vi "Bundle control and indicator references.vi"(8 "error in":errorcluster, 11 "UI elements cluster":T2) -> (0 "error out":errorcluster, 3 "UI elements cluster":T2)   [LabVIEW 2020]
uses:
  Typedefs/UI ctrl refs cluster.ctl
  Typedefs/Laser control knob.ctl
  Typedefs/Frame Size.ctl
  Typedefs/Plane Mode.ctl
  Typedefs/PMT control knob.ctl
  Typedefs/XY Stage_Move.ctl
  Typedefs/test_fpga_control.ctl
  Acquisition/Typedefs/Ref DAQ Param.ctl
  Experiment Type.ctl
  Biology Information.ctl
  Global Variables/gl_UI Ctrl Refs.vi
panel:
  out "Cluster":T1
  in  "RefDAQParam 2":refnum<vi>
  out "Ctrl ref names in typedef cluster":string[](array[string])
  out "Dynamically acquired UI element names":string[](array[string])
  out "Errors":errorcluster[](array[cluster])
  out "UI element names and status":cluster{"Label.Text":string, "Found":bool}[](array[cluster])
  # "<----- If the LED is off for a UI element it means that that this VI fails to acquire its reference correctly. In that case upgrade this VI to handle that element."
  # "The top 5 should be the same.\nThe rest should be updated so not the same."
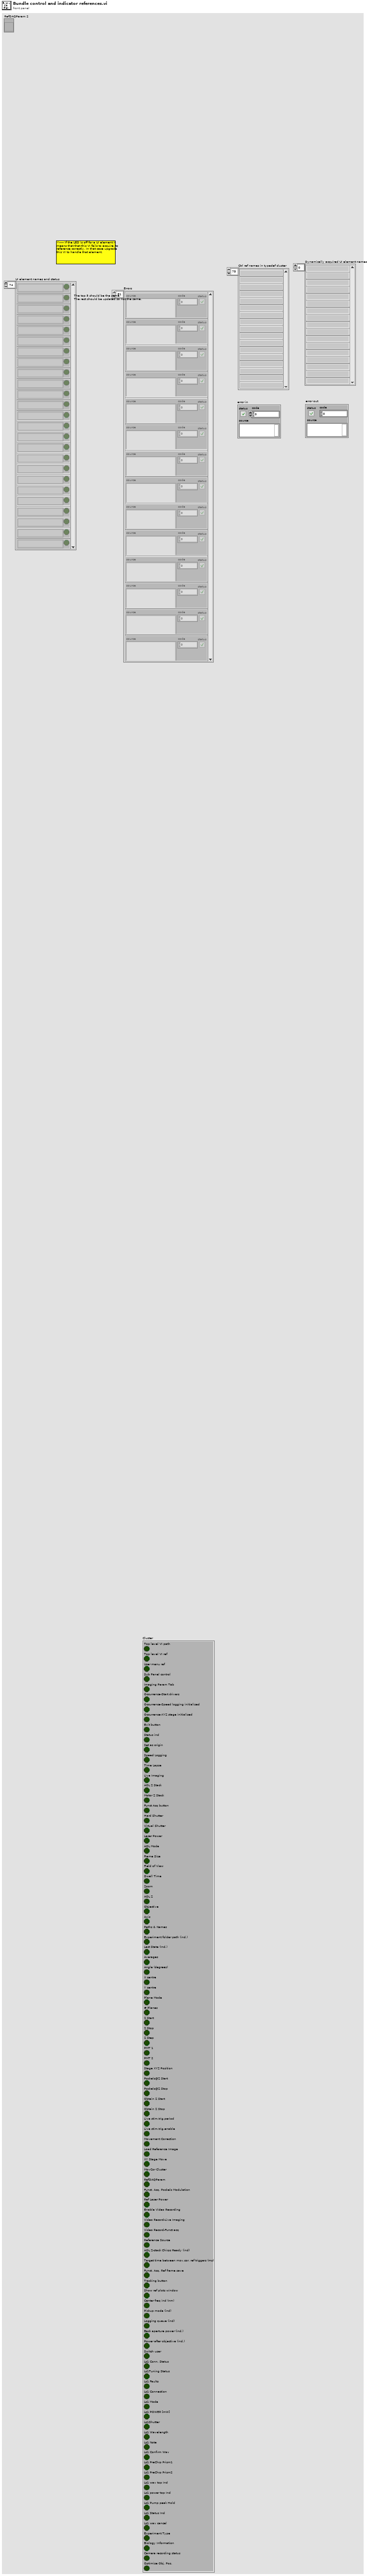
[diagram p1: front panel]
types:
  T1 = cluster{"Top level VI path":bool, "Top level VI ref":bool, "User menu ref":bool, "Sub Panel control":bool, "Imaging Param Tab":bool, "Occurrence-Start drivers":bool, "Occurrence-Speed logging initialised":bool, "Occurrence-XYZ stage initialised":bool, "Exit button":bool, "Status ind":bool, "Set as origin":bool, "Speed Logging":bool, "Time Lapse":bool, "Live Imaging":bool, "AOL Z Stack":bool, "Motor Z Stack":bool, "Funct Acq button":bool, "Hard Shutter":bool, "Virtual Shutter":bool, "Laser Power":bool, "AOL Mode":bool, "Frame Size":bool, "Field of View":bool, "Dwell Time":bool, "Zoom":bool, "AOL Z":bool, "Objective":bool, "Axis":bool, "Paths & Names":bool, "Experiment folder path (ind.)":bool, "Last State (Ind.)":bool, "Averages":bool, "Angle (degrees)":bool, "X centre":bool, "Y centre":bool, "Plane Mode":bool, "# Planes":bool, "Z Start":bool, "Z Stop":bool, "Z Step":bool, "PMT 1":bool, "PMT 2":bool, "Stage XYZ Position":bool, "Pockels@Z Start":bool, "Pockels@Z Stop":bool, "Obtain Z Start":bool, "Obtain Z Stop":bool, "Live stim.trig.period":bool, "Live stim.trig.enable":bool, "Movement Correction":bool, "Load Reference Image":bool, "XY Stage Move":bool, "MovCor Cluster":bool, "RefDAQParam":bool, "Funct. Acq. Pockels Modulation":bool, "Ref Laser Power":bool, "Enable Video Recording":bool, "Video Record-Live Imaging":bool, "Video Record-Funct acq":bool, "Reference Source":bool, "AOL Z-stack Chirps Ready (ind)":bool, "Target time between mov.cor. ref triggers (ms)":bool, "Funct. Acq. Ref frame save":bool, "Tracking button":bool, "Show ref plots window":bool, "Center freq ind (nm)":bool, "Pickup mode (ind)":bool, "Logging queue (ind)":bool, "Back aperture power (ind.)":bool, "Power after objective (ind.)":bool, "Switch user":bool, "Ls1 Conn. Status":bool, "Ls1Tuning Status":bool, "Ls1 Faults":bool, "Ls1 Connection":bool, "Ls1 Mode":bool, "Ls1 POWER [mW]":bool, "Ls1Shutter":bool, "Ls1 Wavelength":bool, "Ls1 Note":bool, "Ls1 Confirm Wav":bool, "Ls1 PreChrp Prism1":bool, "Ls1 PreChrp Prism2":bool, "Ls1 wav top Ind":bool, "Ls1 power top Ind":bool, "Ls1 Pump peak Hold":bool, "Ls1 Status Ind":bool, "Ls1 wav cancel":bool, "Experiment Type":bool, "Biology Information":bool, "Camera recording status":bool, "Optimise Obj. Pos.":bool}
  T2 = typedef "UI ctrl refs cluster.ctl" = cluster{"Top level VI path":path, "Top level VI ref":refnum<vi>, "User menu ref":refnum<k9>, "Sub Panel control":refnum<vi>, "Imaging Param Tab":refnum<vi>, "Occurrence-Start drivers":refnum<k4>, "Occurrence-Speed logging initialised":refnum<k4>, "Occurrence-XYZ stage initialised":refnum<k4>, "Exit button":refnum<vi>, "Status ind":refnum<vi>, "Set as origin":refnum<vi>, "Speed Logging":refnum<vi>, "Time Lapse":refnum<vi>, "Live Imaging":refnum<vi>, "AOL Z Stack":refnum<vi>, "Motor Z Stack":refnum<vi>, "Funct Acq button":refnum<vi>, "Hard Shutter":refnum<vi>, "Virtual Shutter":refnum<vi>, "Laser Power":refnum<vi>, "AOL Mode":refnum<vi>, "Frame Size":refnum<vi>, "Field of View":refnum<vi>, "Dwell Time":refnum<vi>, "Zoom":refnum<vi>, "AOL Z":refnum<vi>, "Objective":refnum<vi>, "Axis":refnum<vi>, "Paths & Names":refnum<vi>, "Experiment folder path (ind.)":refnum<vi>, "Last State (Ind.)":refnum<vi>, "Averages":refnum<vi>, "Angle (degrees)":refnum<vi>, "X centre":refnum<vi>, "Y centre":refnum<vi>, "Plane Mode":refnum<vi>, "# Planes":refnum<vi>, "Z Start":refnum<vi>, "Z Stop":refnum<vi>, "Z Step":refnum<vi>, "PMT 1":refnum<vi>, "PMT 2":refnum<vi>, "Stage XYZ Position":refnum<vi>, "Pockels@Z Start":refnum<vi>, "Pockels@Z Stop":refnum<vi>, "Obtain Z Start":refnum<vi>, "Obtain Z Stop":refnum<vi>, "Live stim.trig.period":refnum<vi>, "Live stim.trig.enable":refnum<vi>, "Movement Correction":refnum<vi>, "Load Reference Image":refnum<vi>, "XY Stage Move":refnum<vi>, "MovCor Cluster":refnum<vi>, "RefDAQParam":refnum<vi>, "Funct. Acq. Pockels Modulation":refnum<vi>, "Ref Laser Power":refnum<vi>, "Enable Video Recording":refnum<vi>, "Video Record-Live Imaging":refnum<vi>, "Video Record-Funct acq":refnum<vi>, "Reference Source":refnum<vi>, "AOL Z-stack Chirps Ready (ind)":refnum<vi>, "Target time between mov.cor. ref triggers (ms)":refnum<vi>, "Funct. Acq. Ref frame save":refnum<vi>, "Tracking button":refnum<vi>, "Show ref plots window":refnum<vi>, "Center freq ind (nm)":refnum<vi>, "Pickup mode (ind)":refnum<vi>, "Logging queue (ind)":refnum<vi>, "Back aperture power (ind.)":refnum<vi>, "Power after objective (ind.)":refnum<vi>, "Switch user":refnum<vi>, "Ls1 Conn. Status":refnum<vi>, "Ls1Tuning Status":refnum<vi>, "Ls1 Faults":refnum<vi>, "Ls1 Connection":refnum<vi>, "Ls1 Mode":refnum<vi>, "Ls1 POWER [mW]":refnum<vi>, "Ls1Shutter":refnum<vi>, "Ls1 Wavelength":refnum<vi>, "Ls1 Note":refnum<vi>, "Ls1 Confirm Wav":refnum<vi>, "Ls1 PreChrp Prism1":refnum<vi>, "Ls1 PreChrp Prism2":refnum<vi>, "Ls1 wav top Ind":refnum<vi>, "Ls1 power top Ind":refnum<vi>, "Ls1 Pump peak Hold":refnum<vi>, "Ls1 Status Ind":refnum<vi>, "Ls1 wav cancel":refnum<vi>, "Experiment Type":refnum<vi>, "Biology Information":refnum<vi>, "Camera recording status":refnum<vi>, "Optimise Obj. Pos.":refnum<vi>}
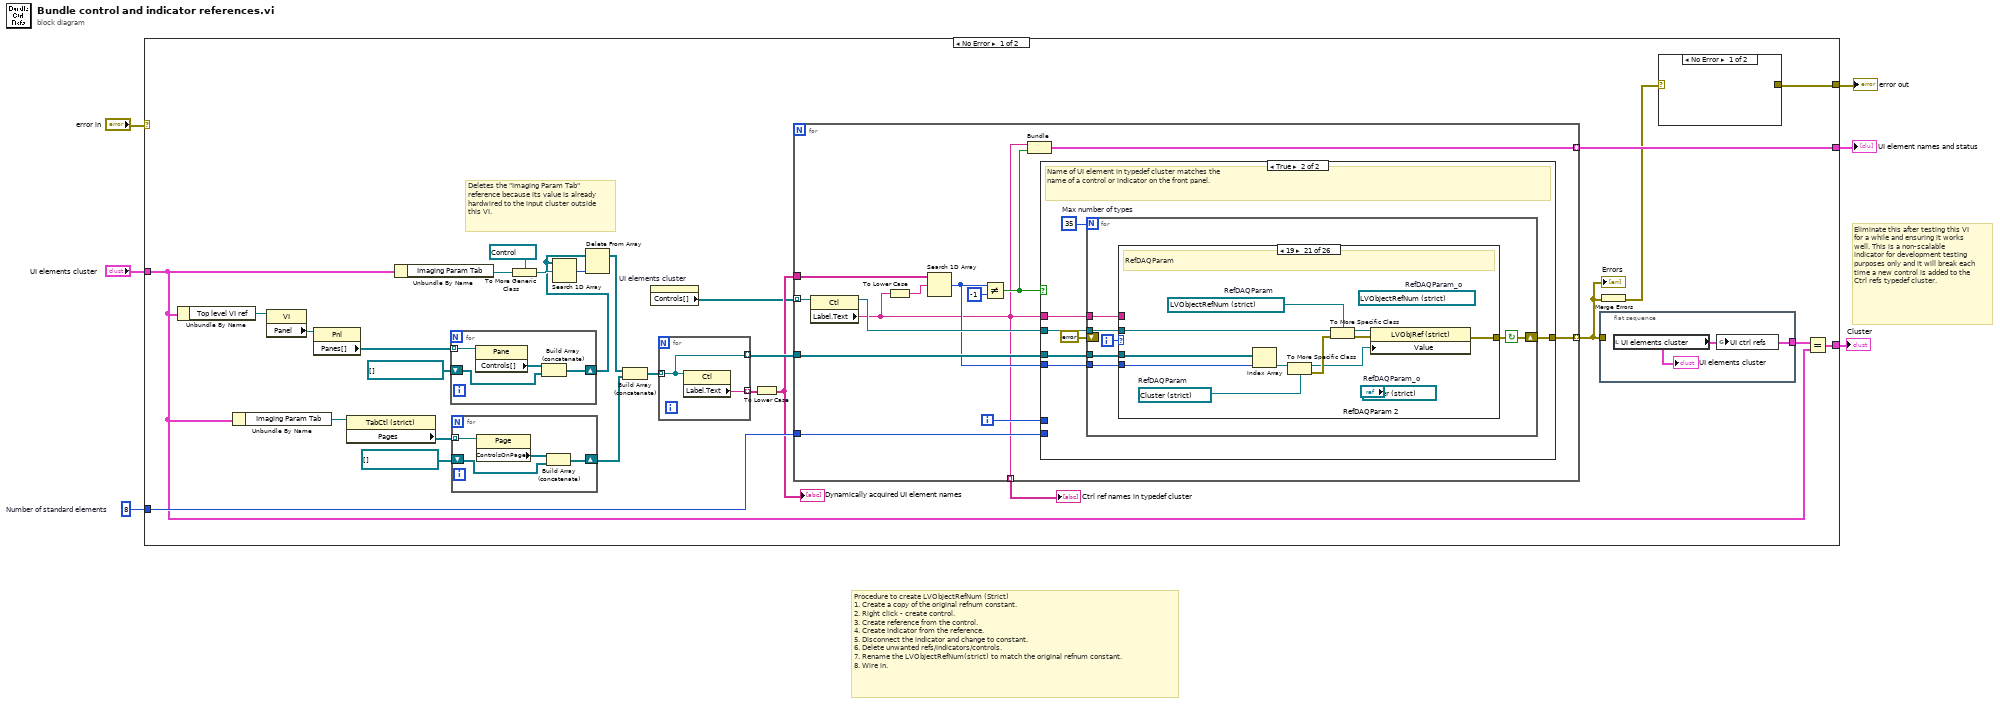
[diagram p0: block diagram]
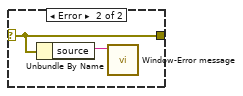
[diagram p2: hidden frame]
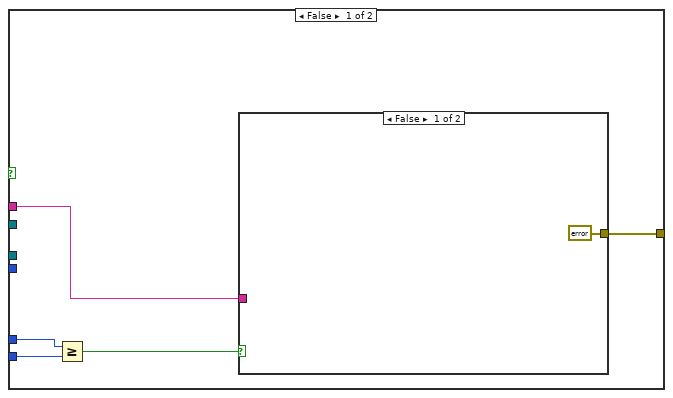
[diagram p3: hidden frame]
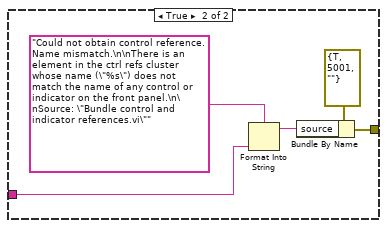
[diagram p4: hidden frame]
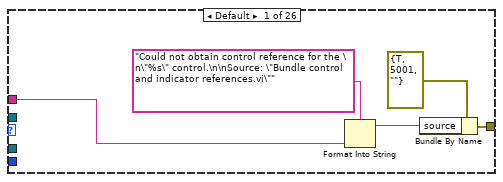
[diagram p5: hidden frame]
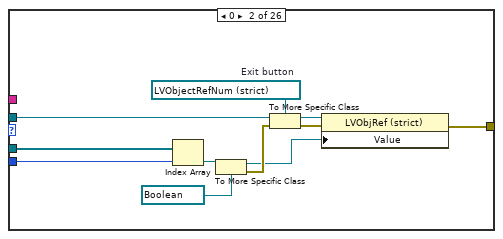
[diagram p6: hidden frame]
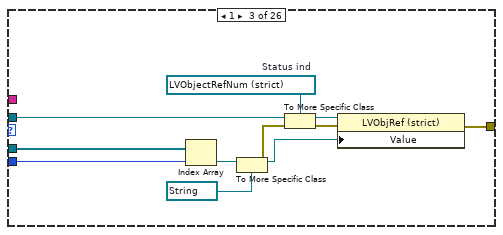
[diagram p7: hidden frame]
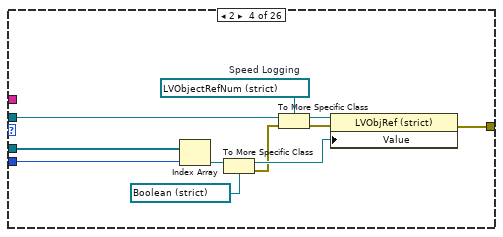
[diagram p8: hidden frame]
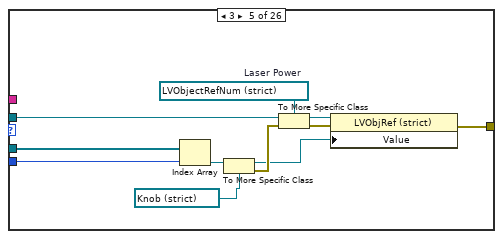
[diagram p9: hidden frame]
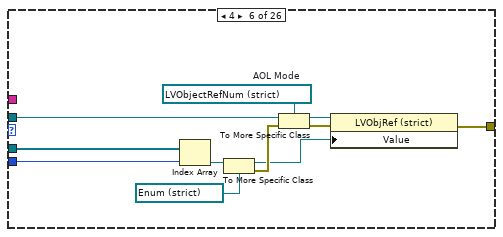
[diagram p10: hidden frame]
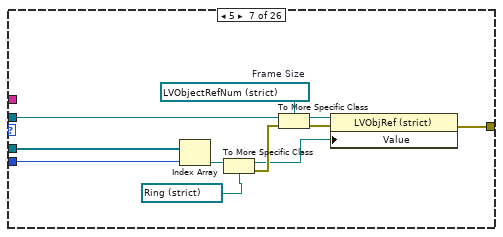
[diagram p11: hidden frame]
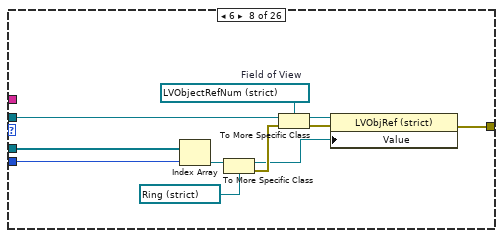
[diagram p12: hidden frame]
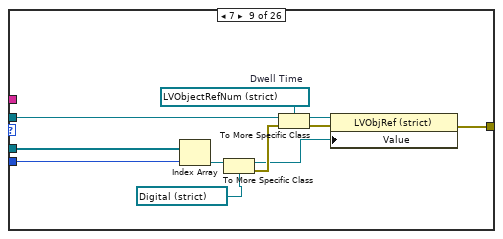
[diagram p13: hidden frame]
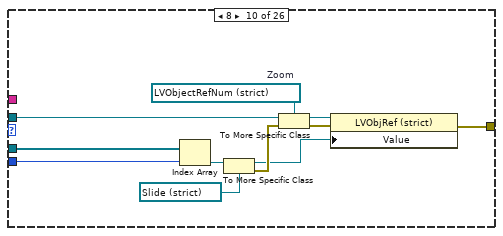
[diagram p14: hidden frame]
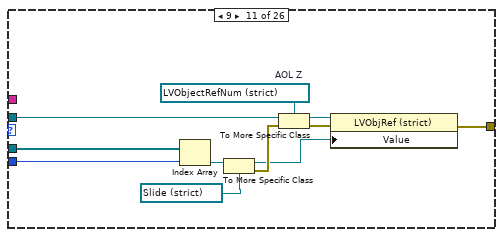
[diagram p15: hidden frame]
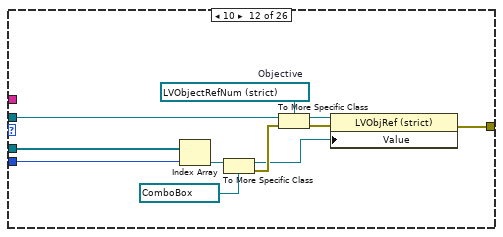
[diagram p16: hidden frame]
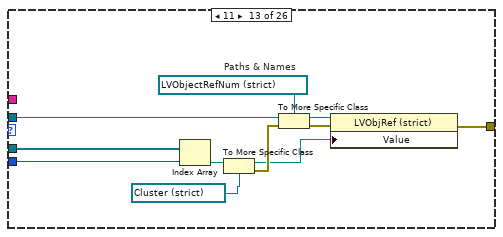
[diagram p17: hidden frame]
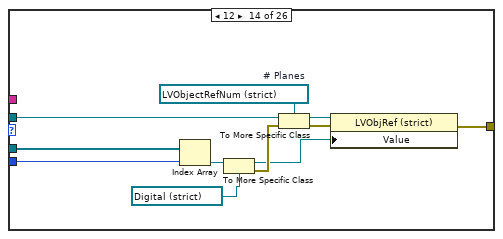
[diagram p18: hidden frame]
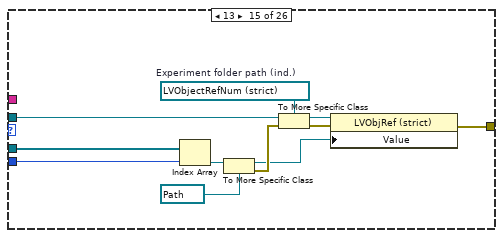
[diagram p19: hidden frame]
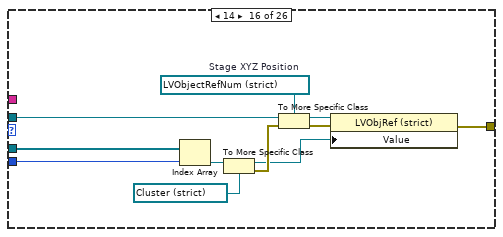
[diagram p20: hidden frame]
diagram:
  w2 = 8  # Number of standard elements
  # "Procedure to create LVObjectRefNum (Strict)\n1. Create a copy of the original refnum constant.\n2. Right click - create control.\n3. Create reference from the control.\n4. Create indicator from the reference.\n5. Disconnect the indicator and change to constant.\n6. Delete unwanted refs/indicators/controls.\n7. Rename the LVObjectRefNum(strict) to match the original refnum constant.\n8. Wire in."
  # "Eliminate this after testing this VI for a while and ensuring it works well. This is a non-scalable indicator for development testing purposes only and it will break each time a new control is added to the Ctrl refs typedef cluster."
  n1 = case shown="No Error" "error in" {
    selector: "error in" -> [_ w365]
    tunnel: [w25 _] -> w6
    tunnel: "UI elements cluster" -> [w11 _]
    tunnel: [w23 _] -> w1
    tunnel: [w14 w365] -> w3
    tunnel: w2 -> [w13 _]
    frame No Error {
      # "Deletes the \"Imaging Param Tab\" reference because its value is already hardwired to the input cluster outside this VI."
      n2 = Unbundle By Name(w11) -> ("Top level VI ref"=w33:refnum<vi>)
      n3 = Unbundle By Name(w11) -> ("Imaging Param Tab"=w20:refnum<vi>)
      n4 = property on="Property Node" class="VI"(reference=w33) -> ("Panel"=w34:refnum<vi>)  [unwired: 1 in, 2 out]
      n5 = property on="Property Node" class="Pnl"(reference=w34) -> ("Panes[]"=w31:refnum<vi>[])  [unwired: 1 in, 2 out]
      n6 = property on="Property Node" class="TabCtl (strict)"(reference=w20) -> ("Pages"=w30:refnum<vi>[])  [unwired: 1 in, 2 out]
      n7 = Unbundle By Name(w11) -> ("Imaging Param Tab"=w12:refnum<vi>)
      n8 = for {
        shift-right: [w363] -> w10
        shift-left: refnum<vi>[] [] -> [w362]
        tunnel: w31 -> [w361] mode=indexing
        n9 = property class="Pane"(reference=w361) -> ("Controls[]"=w364:refnum<vi>[])  [unwired: 1 in, 2 out]
        n10 = Build Array (concatenate)(w364, w362) -> (w363:refnum<vi>[])
      }
      n11 = for {
        shift-right: [w357] -> w28
        shift-left: refnum<vi>[] [] -> [w356]
        tunnel: w30 -> [w355] mode=indexing
        n12 = property class="Page"(reference=w355) -> ("ControlsOnPage"=w358:refnum<vi>[])  [unwired: 1 in, 2 out]
        n13 = Build Array (concatenate)(w358, w356) -> (w357:refnum<vi>[])
      }
      n14 = To More Generic Class(target class=refnum<vi> refnum ("element"), reference=w12) -> (generic class reference=w19:refnum<vi>)
      n15 = Search 1D Array(1D array=w10, element=w19) -> (index of element=w17:i32)  [unwired: 1 in]
      n16 = Delete From Array(array=w10, index=w17) -> (array with subset deleted=w16:refnum<vi>[])  [unwired: 1 in, 1 out]
      n17 = Build Array (concatenate)(w16, w28) -> (w27:refnum<vi>[])
      n18 = property on="UI elements cluster" class="Clust (strict)"() -> ("Controls[]"=w7:refnum<vi>[])  [unwired: 2 in, 2 out]
      n19 = for {
        tunnel: w27 -> [w359] mode=indexing
        tunnel: [w360] -> w26 mode=indexing
        tunnel: [w359] -> w24 mode=indexing
        n20 = property on="Property Node" class="Ctl"(reference=w359) -> ("Label.Text"=w360:string)  [unwired: 1 in, 2 out]
      }
      n21 = To Lower Case(string=w26) -> (all lower case string=w9:string[])
      "Dynamically acquired UI element names" <- w9
      n22 = for {
        tunnel: w7 -> [w50] mode=indexing
        tunnel: w9 -> [w49]
        tunnel: [w47] -> w25 mode=indexing
        tunnel: [w45] -> w22 mode=indexing
        tunnel: w24 -> [w43]
        tunnel: w13 -> [w40]
        tunnel: [w38] -> w8 mode=indexing
        i -> [w41]
        n23 = property on="Property Node" class="Ctl"(reference=w50) -> (reference out=w46:refnum<vi>, "Label.Text"=w38:string)  [unwired: 1 in, 1 out]
        n24 = To Lower Case(string=w38) -> (all lower case string=w42:string)
        n25 = Search 1D Array(1D array=w49, element=w42) -> (index of element=w39:i32)  [unwired: 1 in]
        n26 = Not Equal?(x=w39, y=-1) -> (x != y?=w44:bool)
        n27 = Bundle("Label.Text"=w38, w44) -> (w47:cluster{"Label.Text":string, bool})  [unwired: 1 in]
        n28 = case shown="True" w44 {
          tunnel: w46 -> [_ w68]
          tunnel: [w53 w67] -> w45
          tunnel: w43 -> [_ w66]
          tunnel: w39 -> [_ w65]
          tunnel: w38 -> [w51 w62]
          tunnel: w41 -> [w55 _]
          tunnel: w40 -> [w52 _]
          frame False {
            n29 = Greater Or Equal?(x=w55, y=w52) -> (x >= y?=w54:bool)
            n30 = case shown="False" w54 {
              tunnel: [errorcluster {"status"=FALSE, "code"=0, "source"=""} ("error out") w60] -> w53
              tunnel: w51 -> [_ w57]
              frame False {
              }
              frame True {
                n31 = Format Into String(format string="Could not obtain control reference. Name mismatch.\n\nThere is an element in the ctrl refs cluster whose name (\"%s\") does not match the name of any control or indicator on the front panel.\n\nSource: \"Bundle control and indicator references.vi\"" ("source"), w57) -> (resulting string=w59:string)  [unwired: 2 in, 1 out]
                n32 = Bundle By Name(cluster=errorcluster {"status"=TRUE, "code"=5001, "source"=""} ("error out"), "source"=w59) -> (w60:errorcluster)
              }
            }
          }
          frame True {
            w64 = 35  # Max number of types
            # "Name of UI element in typedef cluster matches the\nname of a control or indicator on the front panel."
            n33 = for {
              N: w64 -> [_]
              tunnel: w68 -> [w74]
              tunnel: w66 -> [w73]
              tunnel: w65 -> [w72]
              shift-right: [w70] -> w67
              shift-left: errorcluster {"status"=FALSE, "code"=0, "source"=""} ("error out") -> [_]
              tunnel: w62 -> [w69]
              i -> [w71]
              stop <- w70 continue-if-true
              n34 = case shown="19" w71 {
                tunnel: w74 -> [_ w86 w101 w112 w123 w134 w145 w156 w167 w178 w189 w200 w211 w222 w233 w244 w255 w266 w277 w288 w299 w310 w321 w332 w343 w349]
                tunnel: [w78 w83 w100 w109 w119 w130 w141 w152 w163 w174 w185 w196 w207 w218 w229 w240 w251 w262 w273 w284 w295 w306 w317 w328 w339 w346] -> w70
                tunnel: w73 -> [_ w84 w99 w111 w122 w133 w144 w155 w166 w177 w188 w199 w210 w221 w232 w243 w254 w265 w276 w287 w298 w309 w320 w331 w342 w348]
                tunnel: w72 -> [_ w85 w98 w110 w121 w132 w143 w154 w165 w176 w187 w198 w209 w220 w231 w242 w253 w264 w275 w286 w297 w308 w319 w330 w341 w347]
                tunnel: w69 -> [w76 _ _ _ _ _ _ _ _ _ _ _ _ _ _ _ _ _ _ _ _ _ _ _ _ _]
                frame Default {
                  n35 = Format Into String(format string="Could not obtain control reference for the \n\"%s\" control.\n\nSource: \"Bundle control and indicator references.vi\"" ("source"), w76) -> (resulting string=w75:string)  [unwired: 2 in, 1 out]
                  n36 = Bundle By Name(cluster=errorcluster {"status"=TRUE, "code"=5001, "source"=""} ("error out"), "source"=w75) -> (w78:errorcluster)
                }
                frame 0 {
                  w80 = refnum<vi> refnum  # Exit button
                  n37 = Index Array(array=w84, index=w85) -> (element=w89:refnum<vi>)
                  n38 = To More Specific Class(target class=refnum<vi> refnum ("Value"), reference=w89) -> (specific class reference=w81:refnum<vi>, error out=w88:errorcluster)  [unwired: 1 in]
                  n39 = To More Specific Class(target class=w80, reference=w86, error in=w88) -> (specific class reference=w90:refnum<vi>, error out=w87:errorcluster)
                  n40 = property on="Property Node" class="LVObjRef (strict)"(reference=w90, error in=w87, "Value"=w81) -> (error out=w83:errorcluster)  [unwired: 1 out]
                }
                frame 1 {
                  w91 = refnum<vi> refnum  # Status ind
                  n41 = Index Array(array=w99, index=w98) -> (element=w96:refnum<vi>)
                  n42 = To More Specific Class(target class=refnum<vi> refnum ("Status ind"), reference=w96) -> (specific class reference=w95:refnum<vi>, error out=w94:errorcluster)  [unwired: 1 in]
                  n43 = To More Specific Class(target class=w91, reference=w101, error in=w94) -> (specific class reference=w97:refnum<vi>, error out=w93:errorcluster)
                  n44 = property on="Property Node" class="LVObjRef (strict)"(reference=w97, error in=w93, "Value"=w95) -> (error out=w100:errorcluster)  [unwired: 1 out]
                }
                frame 2 {
                  w102 = refnum<vi> refnum  # Speed Logging
                  n45 = Index Array(array=w111, index=w110) -> (element=w108:refnum<vi>)
                  n46 = To More Specific Class(target class=refnum<vi> refnum ("Value"), reference=w108) -> (specific class reference=w107:refnum<vi>, error out=w104:errorcluster)  [unwired: 1 in]
                  n47 = To More Specific Class(target class=w102, reference=w112, error in=w104) -> (specific class reference=w106:refnum<vi>, error out=w105:errorcluster)
                  n48 = property on="Property Node" class="LVObjRef (strict)"(reference=w106, error in=w105, "Value"=w107) -> (error out=w109:errorcluster)  [unwired: 1 out]
                }
                frame 3 {
                  w113 = refnum<vi> refnum  # Laser Power
                  n49 = Index Array(array=w122, index=w121) -> (element=w120:refnum<vi>)
                  n50 = To More Specific Class(target class=refnum<vi> refnum ("Value"), reference=w120) -> (specific class reference=w114:refnum<vi>, error out=w116:errorcluster)  [unwired: 1 in]
                  n51 = To More Specific Class(target class=w113, reference=w123, error in=w116) -> (specific class reference=w118:refnum<vi>, error out=w117:errorcluster)
                  n52 = property on="Property Node" class="LVObjRef (strict)"(reference=w118, error in=w117, "Value"=w114) -> (error out=w119:errorcluster)  [unwired: 1 out]
                }
                frame 4 {
                  w124 = refnum<vi> refnum  # AOL Mode
                  n53 = Index Array(array=w133, index=w132) -> (element=w131:refnum<vi>)
                  n54 = To More Specific Class(target class=refnum<vi> refnum ("Value"), reference=w131) -> (specific class reference=w126:refnum<vi>, error out=w127:errorcluster)  [unwired: 1 in]
                  n55 = To More Specific Class(target class=w124, reference=w134, error in=w127) -> (specific class reference=w129:refnum<vi>, error out=w128:errorcluster)
                  n56 = property on="Property Node" class="LVObjRef (strict)"(reference=w129, error in=w128, "Value"=w126) -> (error out=w130:errorcluster)  [unwired: 1 out]
                }
                frame 5 {
                  w135 = refnum<vi> refnum  # Frame Size
                  n57 = Index Array(array=w144, index=w143) -> (element=w142:refnum<vi>)
                  n58 = To More Specific Class(target class=refnum<vi> refnum ("Value"), reference=w142) -> (specific class reference=w136:refnum<vi>, error out=w138:errorcluster)  [unwired: 1 in]
                  n59 = To More Specific Class(target class=w135, reference=w145, error in=w138) -> (specific class reference=w140:refnum<vi>, error out=w139:errorcluster)
                  n60 = property on="Property Node" class="LVObjRef (strict)"(reference=w140, error in=w139, "Value"=w136) -> (error out=w141:errorcluster)  [unwired: 1 out]
                }
                frame 6 {
                  w146 = refnum<vi> refnum  # Field of View
                  n61 = Index Array(array=w155, index=w154) -> (element=w153:refnum<vi>)
                  n62 = To More Specific Class(target class=refnum<vi> refnum ("Value"), reference=w153) -> (specific class reference=w148:refnum<vi>, error out=w149:errorcluster)  [unwired: 1 in]
                  n63 = To More Specific Class(target class=w146, reference=w156, error in=w149) -> (specific class reference=w151:refnum<vi>, error out=w150:errorcluster)
                  n64 = property on="Property Node" class="LVObjRef (strict)"(reference=w151, error in=w150, "Value"=w148) -> (error out=w152:errorcluster)  [unwired: 1 out]
                }
                frame 7 {
                  w157 = refnum<vi> refnum  # Dwell Time
                  n65 = Index Array(array=w166, index=w165) -> (element=w164:refnum<vi>)
                  n66 = To More Specific Class(target class=refnum<vi> refnum ("Value"), reference=w164) -> (specific class reference=w159:refnum<vi>, error out=w160:errorcluster)  [unwired: 1 in]
                  n67 = To More Specific Class(target class=w157, reference=w167, error in=w160) -> (specific class reference=w162:refnum<vi>, error out=w161:errorcluster)
                  n68 = property on="Property Node" class="LVObjRef (strict)"(reference=w162, error in=w161, "Value"=w159) -> (error out=w163:errorcluster)  [unwired: 1 out]
                }
                frame 8 {
                  w168 = refnum<vi> refnum  # Zoom
                  n69 = Index Array(array=w177, index=w176) -> (element=w175:refnum<vi>)
                  n70 = To More Specific Class(target class=refnum<vi> refnum ("Value"), reference=w175) -> (specific class reference=w170:refnum<vi>, error out=w171:errorcluster)  [unwired: 1 in]
                  n71 = To More Specific Class(target class=w168, reference=w178, error in=w171) -> (specific class reference=w173:refnum<vi>, error out=w172:errorcluster)
                  n72 = property on="Property Node" class="LVObjRef (strict)"(reference=w173, error in=w172, "Value"=w170) -> (error out=w174:errorcluster)  [unwired: 1 out]
                }
                frame 9 {
                  w179 = refnum<vi> refnum  # AOL Z
                  n73 = Index Array(array=w188, index=w187) -> (element=w186:refnum<vi>)
                  n74 = To More Specific Class(target class=refnum<vi> refnum ("Value"), reference=w186) -> (specific class reference=w181:refnum<vi>, error out=w182:errorcluster)  [unwired: 1 in]
                  n75 = To More Specific Class(target class=w179, reference=w189, error in=w182) -> (specific class reference=w184:refnum<vi>, error out=w183:errorcluster)
                  n76 = property on="Property Node" class="LVObjRef (strict)"(reference=w184, error in=w183, "Value"=w181) -> (error out=w185:errorcluster)  [unwired: 1 out]
                }
                frame 10 {
                  w190 = refnum<vi> refnum  # Objective
                  n77 = Index Array(array=w199, index=w198) -> (element=w197:refnum<vi>)
                  n78 = To More Specific Class(target class=refnum<vi> refnum ("Value"), reference=w197) -> (specific class reference=w192:refnum<vi>, error out=w193:errorcluster)  [unwired: 1 in]
                  n79 = To More Specific Class(target class=w190, reference=w200, error in=w193) -> (specific class reference=w195:refnum<vi>, error out=w194:errorcluster)
                  n80 = property on="Property Node" class="LVObjRef (strict)"(reference=w195, error in=w194, "Value"=w192) -> (error out=w196:errorcluster)  [unwired: 1 out]
                }
                frame 11 {
                  w202 = refnum<vi> refnum  # Paths & Names
                  n81 = Index Array(array=w210, index=w209) -> (element=w208:refnum<vi>)
                  n82 = To More Specific Class(target class=refnum<vi> refnum ("Paths & Names"), reference=w208) -> (specific class reference=w203:refnum<vi>, error out=w204:errorcluster)  [unwired: 1 in]
                  n83 = To More Specific Class(target class=w202, reference=w211, error in=w204) -> (specific class reference=w206:refnum<vi>, error out=w205:errorcluster)
                  n84 = property on="Property Node" class="LVObjRef (strict)"(reference=w206, error in=w205, "Value"=w203) -> (error out=w207:errorcluster)  [unwired: 1 out]
                }
                frame 12 {
                  w212 = refnum<vi> refnum  # # Planes
                  n85 = Index Array(array=w221, index=w220) -> (element=w219:refnum<vi>)
                  n86 = To More Specific Class(target class=refnum<vi> refnum ("Value"), reference=w219) -> (specific class reference=w214:refnum<vi>, error out=w215:errorcluster)  [unwired: 1 in]
                  n87 = To More Specific Class(target class=w212, reference=w222, error in=w215) -> (specific class reference=w217:refnum<vi>, error out=w216:errorcluster)
                  n88 = property on="Property Node" class="LVObjRef (strict)"(reference=w217, error in=w216, "Value"=w214) -> (error out=w218:errorcluster)  [unwired: 1 out]
                }
                frame 13 {
                  w224 = refnum<vi> refnum  # Experiment folder path (ind.)
                  n89 = Index Array(array=w232, index=w231) -> (element=w230:refnum<vi>)
                  n90 = To More Specific Class(target class=refnum<vi> refnum ("Experiment folder path (ind.)"), reference=w230) -> (specific class reference=w225:refnum<vi>, error out=w226:errorcluster)  [unwired: 1 in]
                  n91 = To More Specific Class(target class=w224, reference=w233, error in=w226) -> (specific class reference=w228:refnum<vi>, error out=w227:errorcluster)
                  n92 = property on="Property Node" class="LVObjRef (strict)"(reference=w228, error in=w227, "Value"=w225) -> (error out=w229:errorcluster)  [unwired: 1 out]
                }
                frame 14 {
                  w234 = refnum<vi> refnum  # Stage XYZ Position
                  n93 = Index Array(array=w243, index=w242) -> (element=w241:refnum<vi>)
                  n94 = To More Specific Class(target class=refnum<vi> refnum ("Value"), reference=w241) -> (specific class reference=w236:refnum<vi>, error out=w237:errorcluster)  [unwired: 1 in]
                  n95 = To More Specific Class(target class=w234, reference=w244, error in=w237) -> (specific class reference=w239:refnum<vi>, error out=w238:errorcluster)
                  n96 = property on="Property Node" class="LVObjRef (strict)"(reference=w239, error in=w238, "Value"=w236) -> (error out=w240:errorcluster)  [unwired: 1 out]
                }
                frame 15 {
                  w245 = refnum<vi> refnum  # Pockels@Z Stop
                  n97 = Index Array(array=w254, index=w253) -> (element=w252:refnum<vi>)
                  n98 = To More Specific Class(target class=refnum<vi> refnum ("Value"), reference=w252) -> (specific class reference=w247:refnum<vi>, error out=w248:errorcluster)  [unwired: 1 in]
                  n99 = To More Specific Class(target class=w245, reference=w255, error in=w248) -> (specific class reference=w250:refnum<vi>, error out=w249:errorcluster)
                  n100 = property on="Property Node" class="LVObjRef (strict)"(reference=w250, error in=w249, "Value"=w247) -> (error out=w251:errorcluster)  [unwired: 1 out]
                }
                frame 16 {
                  w256 = refnum<vi> refnum  # Obtain Z Stop
                  n101 = Index Array(array=w265, index=w264) -> (element=w263:refnum<vi>)
                  n102 = To More Specific Class(target class=refnum<vi> refnum ("Value"), reference=w263) -> (specific class reference=w257:refnum<vi>, error out=w259:errorcluster)  [unwired: 1 in]
                  n103 = To More Specific Class(target class=w256, reference=w266, error in=w259) -> (specific class reference=w261:refnum<vi>, error out=w260:errorcluster)
                  n104 = property on="Property Node" class="LVObjRef (strict)"(reference=w261, error in=w260, "Value"=w257) -> (error out=w262:errorcluster)  [unwired: 1 out]
                }
                frame 17 {
                  w267 = refnum<vi> refnum  # XY Stage Move
                  # "XY Stage Move"
                  n105 = Index Array(array=w276, index=w275) -> (element=w274:refnum<vi>)
                  n106 = To More Specific Class(target class=refnum<vi> refnum ("XY Stage Move"), reference=w274) -> (specific class reference=w269:refnum<vi>, error out=w270:errorcluster)  [unwired: 1 in]
                  n107 = To More Specific Class(target class=w267, reference=w277, error in=w270) -> (specific class reference=w272:refnum<vi>, error out=w271:errorcluster)
                  n108 = property on="Property Node" class="LVObjRef (strict)"(reference=w272, error in=w271, "Value"=w269) -> (error out=w273:errorcluster)  [unwired: 1 out]
                }
                frame 18 {
                  w278 = refnum<vi> refnum  # MovCor Cluster
                  w279 = refnum<vi> refnum  # MovCor Cluster
                  # "MovCor Cluster"
                  n109 = Index Array(array=w287, index=w286) -> (element=w285:refnum<vi>)
                  n110 = To More Specific Class(target class=w278, reference=w285) -> (specific class reference=w280:refnum<vi>, error out=w281:errorcluster)  [unwired: 1 in]
                  n111 = To More Specific Class(target class=w279, reference=w288, error in=w281) -> (specific class reference=w283:refnum<vi>, error out=w282:errorcluster)
                  n112 = property on="Property Node" class="LVObjRef (strict)"(reference=w283, error in=w282, "Value"=w280) -> (error out=w284:errorcluster)  [unwired: 1 out]
                }
                frame 19 {
                  w289 = refnum<vi> refnum  # RefDAQParam
                  w290 = refnum<vi> refnum  # RefDAQParam
                  (unwired) refnum<vi> refnum  # RefDAQParam_o
                  (unwired) refnum<vi> refnum  # RefDAQParam_o
                  # "RefDAQParam"
                  n113 = Index Array(array=w298, index=w297) -> (element=w296:refnum<vi>)
                  n114 = To More Specific Class(target class=w289, reference=w296) -> (specific class reference=w291:refnum<vi>, error out=w292:errorcluster)  [unwired: 1 in]
                  n115 = To More Specific Class(target class=w290, reference=w299, error in=w292) -> (specific class reference=w294:refnum<vi>, error out=w293:errorcluster)
                  n116 = property on="Property Node" class="LVObjRef (strict)"(reference=w294, error in=w293, "Value"=w291) -> (error out=w295:errorcluster)  [unwired: 1 out]
                }
                frame 20 {
                  w300 = refnum<vi> refnum  # Ref Laser Power
                  n117 = Index Array(array=w309, index=w308) -> (element=w307:refnum<vi>)
                  n118 = To More Specific Class(target class=refnum<vi> refnum ("Ref Laser Power"), reference=w307) -> (specific class reference=w302:refnum<vi>, error out=w303:errorcluster)  [unwired: 1 in]
                  n119 = To More Specific Class(target class=w300, reference=w310, error in=w303) -> (specific class reference=w305:refnum<vi>, error out=w304:errorcluster)
                  n120 = property on="Property Node" class="LVObjRef (strict)"(reference=w305, error in=w304, "Value"=w302) -> (error out=w306:errorcluster)  [unwired: 1 out]
                }
                frame 21 {
                  w311 = refnum<vi> refnum  # Reference Source
                  n121 = Index Array(array=w320, index=w319) -> (element=w318:refnum<vi>)
                  n122 = To More Specific Class(target class=refnum<vi> refnum ("Reference Source"), reference=w318) -> (specific class reference=w313:refnum<vi>, error out=w314:errorcluster)  [unwired: 1 in]
                  n123 = To More Specific Class(target class=w311, reference=w321, error in=w314) -> (specific class reference=w316:refnum<vi>, error out=w315:errorcluster)
                  n124 = property on="Property Node" class="LVObjRef (strict)"(reference=w316, error in=w315, "Value"=w313) -> (error out=w317:errorcluster)  [unwired: 1 out]
                }
                frame 22 {
                  w322 = refnum<vi> refnum  # Experiment Type
                  w323 = refnum<vi> refnum  # Experiment Type
                  n125 = Index Array(array=w331, index=w330) -> (element=w329:refnum<vi>)
                  n126 = To More Specific Class(target class=w323, reference=w329) -> (specific class reference=w324:refnum<vi>, error out=w325:errorcluster)  [unwired: 1 in]
                  n127 = To More Specific Class(target class=w322, reference=w332, error in=w325) -> (specific class reference=w327:refnum<vi>, error out=w326:errorcluster)
                  n128 = property on="Property Node" class="LVObjRef (strict)"(reference=w327, error in=w326, "Value"=w324) -> (error out=w328:errorcluster)  [unwired: 1 out]
                }
                frame 23 {
                  w333 = refnum<vi> refnum  # Biology Information
                  w334 = refnum<vi> refnum  # Biology Information
                  n129 = Index Array(array=w342, index=w341) -> (element=w340:refnum<vi>)
                  n130 = To More Specific Class(target class=w333, reference=w340) -> (specific class reference=w335:refnum<vi>, error out=w336:errorcluster)  [unwired: 1 in]
                  n131 = To More Specific Class(target class=w334, reference=w343, error in=w336) -> (specific class reference=w338:refnum<vi>, error out=w337:errorcluster)
                  n132 = property on="Property Node" class="LVObjRef (strict)"(reference=w338, error in=w337, "Value"=w335) -> (error out=w339:errorcluster)  [unwired: 1 out]
                }
                frame 24 {
                  w344 = refnum<vi> refnum  # Optimise Obj. Pos.
                  w345 = refnum<vi> refnum  # Optimise Obj. Pos.
                  n133 = Index Array(array=w348, index=w347) -> (element=w354:refnum<vi>)
                  n134 = To More Specific Class(target class=w345, reference=w354) -> (specific class reference=w350:refnum<vi>, error out=w351:errorcluster)  [unwired: 1 in]
                  n135 = To More Specific Class(target class=w344, reference=w349, error in=w351) -> (specific class reference=w353:refnum<vi>, error out=w352:errorcluster)
                  n136 = property on="Property Node" class="LVObjRef (strict)"(reference=w353, error in=w352, "Value"=w350) -> (error out=w346:errorcluster)  [unwired: 1 out]
                }
              }
            }
          }
        }
      }
      "Errors" <- w22
      "Ctrl ref names in typedef cluster" <- w8
      n137 = flat-sequence {
        tunnel: w22 -> [_]
        tunnel: [w37] -> w21
        frame #0 {
          n138 = local read "UI elements cluster"() -> (w37:T2)
          "UI elements cluster" <- w37
          n139 = global write "gl_UI Ctrl Refs.vi" "UI ctrl refs"(w37) -> ()
        }
      }
      n140 = Merge Errors(w22) -> (w15:errorcluster)
      n141 = case shown="No Error" w15 {
        selector: w15 -> [_ w36]
        tunnel: [_ w36] -> w14
        frame No Error {
        }
        frame Error {
          n142 = Unbundle By Name(w36) -> ("source"=w35:string)
          n143 = call "Window-Error message.vi"("Message"=w35) -> ()  [unwired: 10 in, 1 out]
        }
      }
      n144 = Equal?(x=w21, y=w11) -> (x = y?=w23:T1)
    }
    frame Error {
    }
  }
  "error out" <- w3
  "UI element names and status" <- w6
  "Cluster" <- w1
